vi "Test citire I2C.vi"() -> ()   [LabVIEW 2020]
uses:
  MCP2221A LabVIEW library/Microchip MCP2221A_64bit/VIs/Private/mcp2221_dll_um_x64.dll
panel:
  out "FRM":i32=3
  out "12 bit temp (C)":dbl=27.2
  out "12 bit Field value (mT) Z":dbl=0.098
  out "12 bit Field value (mT) Y":dbl=0.196
  out "12 bit Field value (mT) X":dbl=0.392
  out "hex integer string":string[](array[string])=["0", "0", "0", "1C", "13", "20", "55", "7", "4", "20"]
  out "i2cRxData out":u8[](array[numeric])=[0, 0, 0, 28, 19, 32, 85, 7, 4, 32]
  in  "use7bitAddress":bool
  in  "slaveAddress":u8=189 format="%.0b"
  in  "bytesToRead":u32=10
  out "handle out":u64=57196
  out "noOfDevs out":u32=1
  in  "error in (no error)":errorcluster
  out "error out":errorcluster
  # "I2C Read Config"
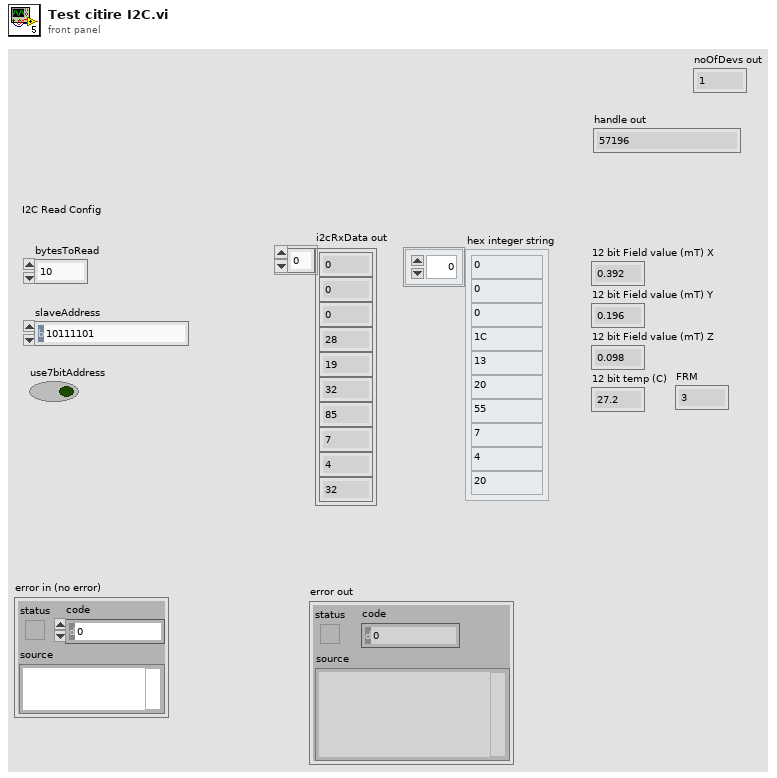
[diagram p1: front panel]
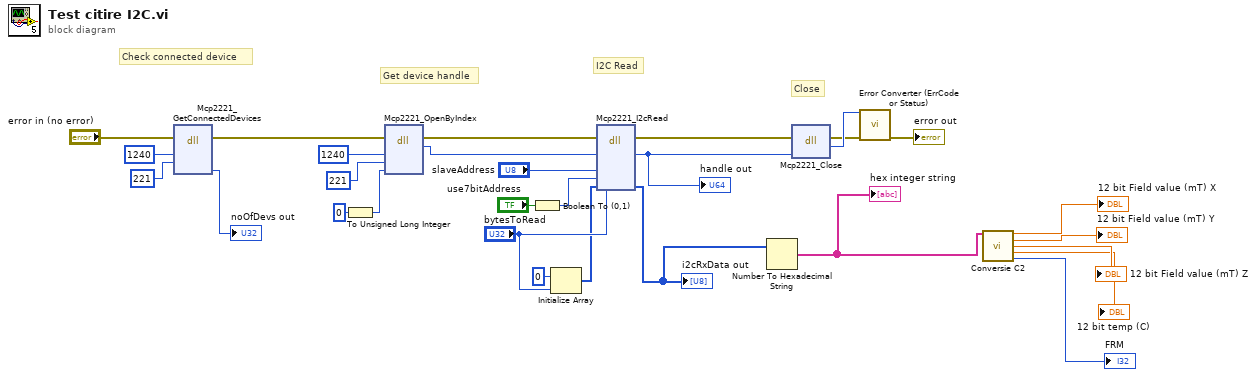
[diagram p0: block diagram]
diagram:
  # "Close"
  # "I2C Read"
  # "Get device handle"
  # "Check connected device"
  n1 = dll-call lib="C:/Users/tuguialexand/Desktop/Licenta/MCP2221A LabVIEW library/Microchip MCP2221A_64bit/VIs/Private/mcp2221_dll_um_x64.dll" fn="Mcp2221_GetConnectedDevices"(error in="error in (no error)", "vid"=u32 1240, "pid"=u32 221) -> (error out=w14:errorcluster, "noOfDevs"=→"noOfDevs out":u32)  [unwired: 6 in, 1 out]
  n2 = To Unsigned Long Integer(number=0 ("index")) -> (unsigned 32bit integer=w17:u32)
  n3 = dll-call lib="C:/Users/tuguialexand/Desktop/Licenta/MCP2221A LabVIEW library/Microchip MCP2221A_64bit/VIs/Private/mcp2221_dll_um_x64.dll" fn="Mcp2221_OpenByIndex"(error in=w14, "VID"=u32 1240, "PID"=u32 221, "index"=w17) -> (error out=w12:errorcluster, "return type"=w13:u64)  [unwired: 5 in, 1 out]
  n4 = Boolean To (0,1)(Boolean="use7bitAddress") -> (0, 1=w23:i16)
  n5 = Initialize Array(u8 0, "bytesToRead") -> (w20:u8[])
  n6 = dll-call lib="C:/Users/tuguialexand/Desktop/Licenta/MCP2221A LabVIEW library/Microchip MCP2221A_64bit/VIs/Private/mcp2221_dll_um_x64.dll" fn="Mcp2221_I2cRead"(error in=w12, "handle"=w13, "bytesToRead"="bytesToRead", "slaveAddress"="slaveAddress", "use7bitAddress"=w23, "i2cRxData"=w20) -> (error out=w8:errorcluster, "handle"=w11:u64, "i2cRxData"=w7:u8[])  [unwired: 6 in, 1 out]
  "handle out" <- w11
  "i2cRxData out" <- w7
  n7 = Number To Hexadecimal String(2:w7) -> (0:w6:string[])  [unwired: 1 in]
  "hex integer string" <- w6
  n8 = dll-call lib="C:/Users/tuguialexand/Desktop/Licenta/MCP2221A LabVIEW library/Microchip MCP2221A_64bit/VIs/Private/mcp2221_dll_um_x64.dll" fn="Mcp2221_Close"(error in=w8, "handle"=w11) -> (error out=w9:errorcluster, "return type"=w10:i32)  [unwired: 3 in, 1 out]
  n9 = call "Error Converter (ErrCode or Status).vi"("error code"=w10, "error in (no error)"=w9) -> ("error out"=→"error out":errorcluster)  [unwired: 13 in]
  n10 = call "Conversie C2.vi"("Array"=w6) -> ("12 bit Field value (mT) X"=→"12 bit Field value (mT) X":dbl, "12 bit Field value (mT) Y"=→"12 bit Field value (mT) Y":dbl, "12 bit Field value (mT) Z"=→"12 bit Field value (mT) Z":dbl, "12 bit temp (C)"=→"12 bit temp (C)":dbl, "FRM"=→"FRM":i32)  [unwired: 10 in]
